vi "Get DI Data from local Daq Q.vi"(8 "error in":errorcluster, 11 "daqThread DI local Q":refnum<queue>) -> (0 "error out":errorcluster, 1 "timestamp":dbl, 2 "data":bool[](array[boolean]), 3 "daqThread DI local Q":refnum<queue>)   [LabVIEW 2017, in "DAQ.lvclass"]
doc: "Developed by Kevin Thompson\nkevin@thompsonengineering.net\n\nCopyright 2018-2020\nThompson Engineering, LLC"
uses:
  DAQ.lvclass
  TD local raw DI Data--cluster.ctl
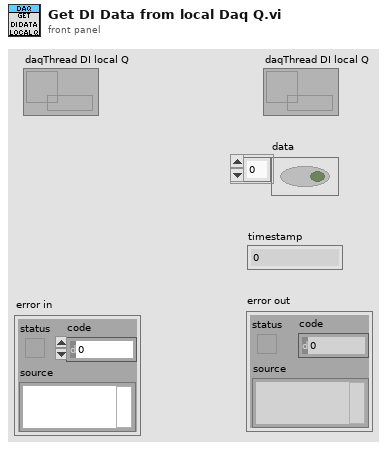
[diagram p1: front panel]
types:
  T1 = typedef "DAQ.lvclass/TD local raw DI Data--cluster.ctl" = cluster{dbl, "data":bool[]}
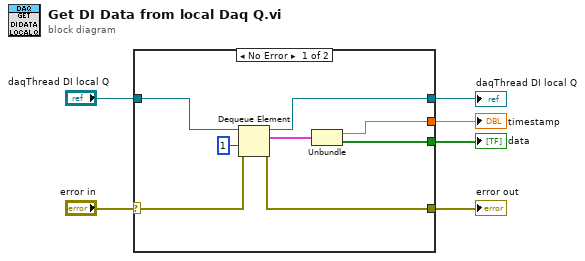
[diagram p0: block diagram]
diagram:
  n1 = case shown="No Error" "error in" {
    selector: "error in" -> [w7 w15]
    tunnel: "daqThread DI local Q" -> [w14 w16]
    tunnel: [w12 _] -> w5
    tunnel: [w11 _] -> w1
    tunnel: [w9 w15] -> w4
    tunnel: [w8 w16] -> w3
    frame No Error {
      n2 = Dequeue Element(queue=w14, timeout in ms (-1)=1, error in (no error)=w7) -> (queue out=w8:refnum<queue>, element=w13:T1, error out=w9:errorcluster)  [unwired: 1 out]
      n3 = Unbundle(w13) -> (w12:dbl, "data"=w11:bool[])
    }
    frame Error {
    }
  }
  "error out" <- w4
  "data" <- w1
  "timestamp" <- w5
  "daqThread DI local Q" <- w3
